vi "Device Change To SetList.vi"(0 "Device List in":refnum<class "Device.lvclass">[](array[class]), 1 "Layout ref":refnum<vi>, 2 "Table History ref":refnum<vi>, 5 "Table Ref In":refnum<vi>, 7 "Dev Index":i32, 9 "Col array in":refnum<class "Column.lvclass">[](array[class]), 11 "DevNums In":i32[](array[numeric])) -> (6 "Table Ref Out":refnum<vi>, 8 "Col. Changes Made?":bool, 10 "Col array out":refnum<class "Column.lvclass">[](array[class]), 15 "DevNums Out":i32[](array[numeric]))   [LabVIEW 2013]
doc: "Push changes in a device back to the SetList table and column array.\nTo delete a device, pass device with empty device col array and empty data table.\nTo resize # of device columns, resize the device col array and add device data to match in size. If the device data doesn't match, data columns will be added or removed as needed without regard to sensible data!"
uses:
  Device/Device.lvclass
  ColumnVIs/Column/Column.lvclass
  TypeDefs/TableHistory.ctl
  TypeDefs/TableArray.ctl
  Master Device/Master Device.lvclass
panel:
  out "Col Length":i32
  out "Index Start":i32
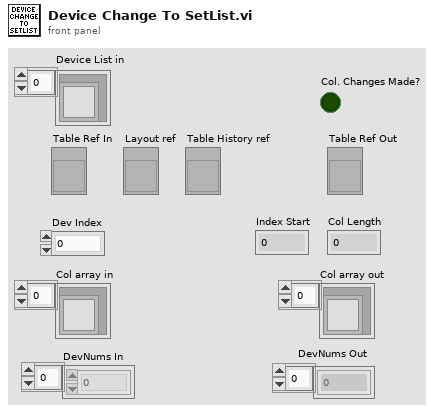
[diagram p1: front panel]
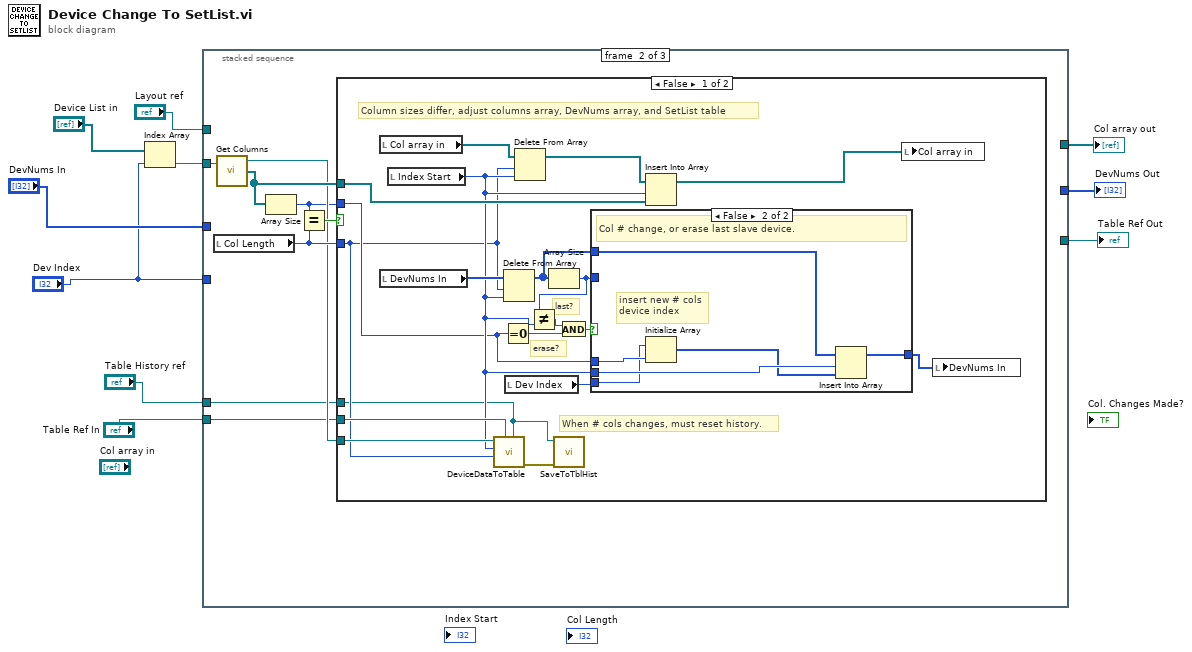
[diagram p0: block diagram]
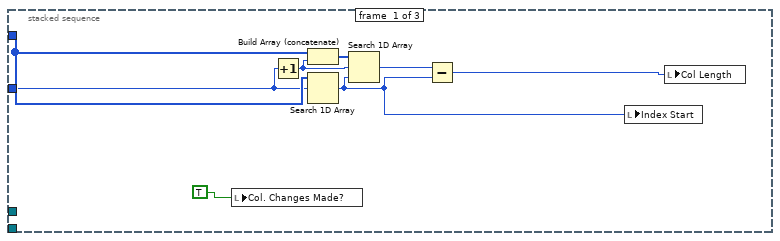
[diagram p2: hidden frame]
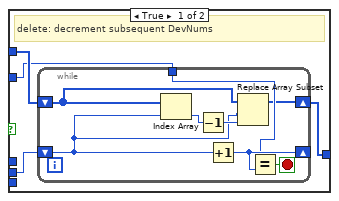
[diagram p3: hidden frame]
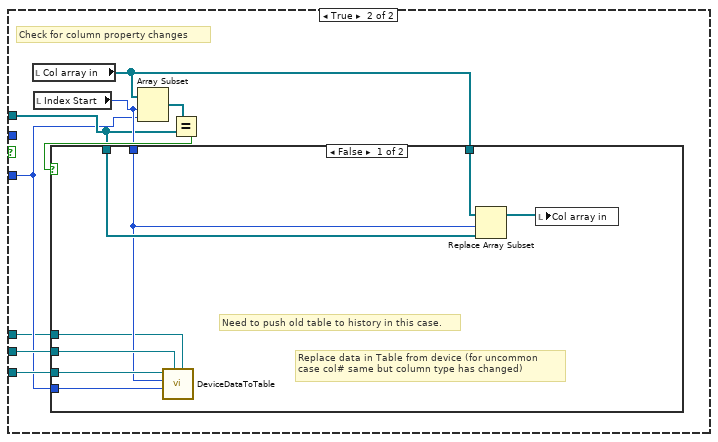
[diagram p4: hidden frame]
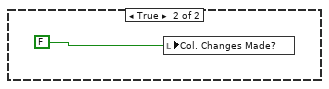
[diagram p5: hidden frame]
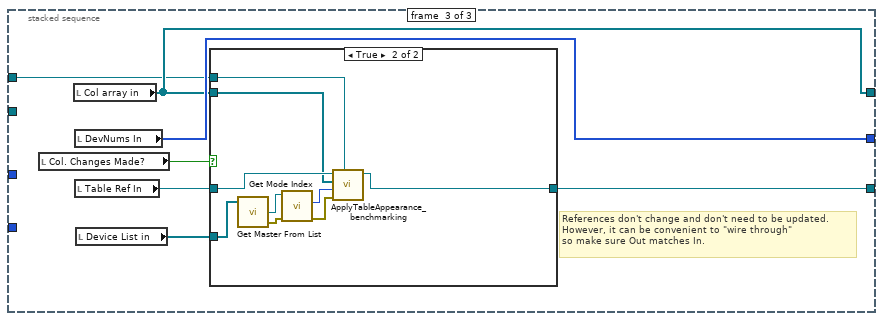
[diagram p6: hidden frame]
diagram:
  n1 = Index Array(array="Device List in", index="Dev Index") -> (element=w7:refnum<class "Device.lvclass">)
  n2 = stacked-sequence {
    tunnel: "DevNums In" -> [w15 _ _]
    tunnel: "Dev Index" -> [w14 _ _]
    tunnel: w7 -> [_ w26 _]
    tunnel: [_ _ w85] -> w6
    tunnel: [_ _ w84] -> w5
    tunnel: [_ _ w83] -> w4
    tunnel: "Layout ref" -> [_ _ w82]
    tunnel: "Table Ref In" -> [_ w20 _]
    tunnel: "Table History ref" -> [_ w19 _]
    frame #0 {
      n3 = local write "Col. Changes Made?"(TRUE) -> ()
      n4 = Increment(x=w14) -> (x+1=w16:i32)
      n5 = Build Array (concatenate)(w15, w16) -> (w17:i32[])
      n6 = Search 1D Array(1D array=w15, element=w14) -> (index of element=w13:i32)  [unwired: 1 in]
      n7 = Search 1D Array(1D array=w17, element=w16, start index (0)=w13) -> (index of element=w18:i32)
      n8 = Subtract(x=w18, y=w13) -> (x-y=w12:i32)
      n9 = local write "Index Start"(w13) -> ()
      n10 = local write "Col Length"(w12) -> ()
    }
    frame #1 {
      n11 = local read "Col Length"() -> (w23:i32)
      n12 = call-dynamic "Get Columns.vi"("Device in"=w26) -> ("Device out"=w22:refnum<class "Device.lvclass">, "Columns"=w24:refnum<class "Column.lvclass">[])  [unwired: 1 in, 1 out]
      n13 = Array Size(array=w24) -> (size(s)=w21:i32)
      n14 = Equal?(x=w21, y=w23) -> (x = y?=w25:bool)
      n15 = case shown="False" w25 {
        tunnel: w24 -> [w43 w68]
        tunnel: w23 -> [w29 w65]
        tunnel: w22 -> [w33 w66]
        tunnel: w21 -> [w30 _]
        tunnel: w20 -> [w32 w67]
        tunnel: w19 -> [w27 w64]
        frame False {
          # "When # cols changes, must reset history."
          # "erase?"
          # "last?"
          # "Column sizes differ, adjust columns array, DevNums array, and SetList table"
          n16 = local read "Col array in"() -> (w45:refnum<class "Column.lvclass">[])
          n17 = local read "DevNums In"() -> (w41:i32[])
          n18 = local read "Index Start"() -> (w31:i32)
          n19 = call "DeviceDataToTable.vi"("Table History ref"=w27, "Table Ref In"=w32, "Col Length"=w29, "Index Start"=w31, "Device object"=w33) -> ("error out"=w28:errorcluster)  [unwired: 6 in]
          n20 = Equal To 0?(x=w30) -> (x = 0?=w35:bool)
          n21 = Delete From Array(array=w41, length=w29, index=w31) -> (array with subset deleted=w37:i32[])  [unwired: 1 out]
          n22 = local read "Dev Index"() -> (w40:i32)
          n23 = Delete From Array "Delete From Array"(array=w45, length=w29, index=w31) -> (array with subset deleted=w44:refnum<class "Column.lvclass">[])  [unwired: 1 out]
          n24 = Array Size(array=w37) -> (size(s)=w36:i32)
          n25 = Not Equal?(x=w36, y=w31) -> (x != y?=w34:bool)
          n26 = call "SaveToTblHist.vi"("error in (no error)"=w28, "Table History ref"=w27) -> ()  [unwired: 9 in, 1 out]
          n27 = And(x=w34, y=w35) -> (x .and. y?=w38:bool)
          n28 = case shown="False" w38 {
            tunnel: w37 -> [w48 w63]
            tunnel: w40 -> [_ w59]
            tunnel: [w46 w62] -> w39
            tunnel: w31 -> [w49 w61]
            tunnel: w36 -> [w47 _]
            tunnel: w30 -> [_ w60]
            frame True {
              # "delete: decrement subsequent DevNums"
              n29 = while {
                tunnel: w47 -> [w51]
                shift-right: [w55] -> _
                shift-left: w49 -> [w53]
                shift-right: [w50] -> w46
                shift-left: w48 -> [w52]
                stop <- w57 stop-if-true
                n30 = Index Array(array=w52, index=w53) -> (element=w56:i32)
                n31 = Decrement(x=w56) -> (x-1=w54:i32)
                n32 = Increment(x=w53) -> (x+1=w55:i32)
                n33 = Replace Array Subset(array=w52, new element=w54, index=w53) -> (w50:i32[])
                n34 = Equal?(x=w51, y=w55) -> (x = y?=w57:bool)
              }
            }
            frame False {
              # "insert new # cols\ndevice index"
              # "Col # change, or erase last slave device."
              n35 = Initialize Array(w59, w60) -> (w58:i32[])
              n36 = Insert Into Array(array=w63, index=w61, new element=w58) -> (w62:i32[])
            }
          }
          n37 = Insert Into Array "Insert Into Array"(array=w44, index=w31, new element=w43) -> (w42:refnum<class "Column.lvclass">[])
          n38 = local write "Col array in"(w42) -> ()
          n39 = local write "DevNums In"(w39) -> ()
        }
        frame True {
          # "Check for column property changes"
          n40 = local read "Col array in"() -> (w70:refnum<class "Column.lvclass">[])
          n41 = local read "Index Start"() -> (w69:i32)
          n42 = Array Subset "Array Subset"(array=w70, index=w69, length=w65) -> (w72:refnum<class "Column.lvclass">[])
          n43 = Equal?(x=w72, y=w68) -> (x = y?=w71:bool)
          n44 = case shown="False" w71 {
            tunnel: w70 -> [w79 _]
            tunnel: w69 -> [w74 _]
            tunnel: w68 -> [w78 _]
            tunnel: w67 -> [w76 _]
            tunnel: w66 -> [w77 _]
            tunnel: w65 -> [w75 _]
            tunnel: w64 -> [w73 _]
            frame False {
              # "Need to push old table to history in this case."
              # "Replace data in Table from device (for uncommon\ncase col# same but column type has changed)"
              n45 = call "DeviceDataToTable.vi"("Table History ref"=w73, "Table Ref In"=w76, "Col Length"=w75, "Index Start"=w74, "Device object"=w77) -> ()  [unwired: 6 in, 1 out]
              n46 = Replace Array Subset "Replace Array Subset"(array=w79, new element=w78, index=w74) -> (w80:refnum<class "Column.lvclass">[])
              n47 = local write "Col array in"(w80) -> ()
            }
            frame True {
              n48 = local write "Col. Changes Made?"(FALSE) -> ()
            }
          }
        }
      }
    }
    frame #2 {
      # "References don't change and don't need to be updated.\nHowever, it can be convenient to \"wire through\"\nso make sure Out matches In."
      n49 = local read "Col. Changes Made?"() -> (w88:bool)
      n50 = local read "Col array in"() -> (w84:refnum<class "Column.lvclass">[])
      n51 = local read "DevNums In"() -> (w85:i32[])
      n52 = local read "Table Ref In"() -> (w87:refnum<vi>)
      n53 = local read "Device List in"() -> (w86:refnum<class "Device.lvclass">[])
      n54 = case shown="True" w88 {
        tunnel: w87 -> [w89 w98]
        tunnel: w84 -> [_ w97]
        tunnel: w86 -> [_ w96]
        tunnel: [w89 w93] -> w83
        tunnel: w82 -> [_ w90]
        frame False {
        }
        frame True {
          n55 = call "Get Master From List.vi"("Device List in"=w96) -> ("error out"=w92:errorcluster, "Master Device"=w95:refnum<class "Master Device.lvclass">)  [unwired: 2 in, 1 out]
          n56 = call-dynamic "Get Mode Index.vi"("error in (no error)"=w92, "Master Device in"=w95) -> ("error out"=w91:errorcluster, "Mode Col"=w94:i32)  [unwired: 7 in, 1 out]
          n57 = call "ApplyTableAppearance_benchmarking.vi"("Layout Ring Ref"=w90, "error in (no error)"=w91, "Mode Index"=w94, "Col Array in"=w97, "Table Ref in"=w98) -> ("Table Ref out"=w93:refnum<vi>)  [unwired: 5 in, 1 out]
        }
      }
    }
  }
  "Table Ref Out" <- w4
  "DevNums Out" <- w6
  "Col array out" <- w5
